vi "Random_Noise.vi"(9 "min":dbl, 10 "max":dbl, 11 "samples":i32) -> (3 "Random Noise":dbl[](array[numeric]))   [LabVIEW 2011]
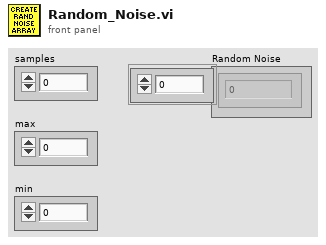
[diagram p1: front panel]
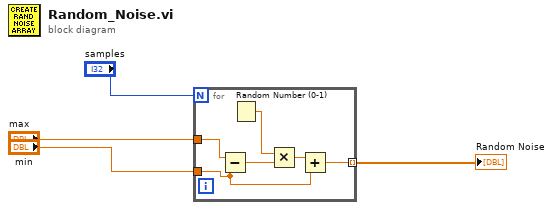
[diagram p0: block diagram]
diagram:
  n1 = for {
    N: "samples" -> [_]
    tunnel: "max" -> [w7]
    tunnel: "min" -> [w6]
    tunnel: [w5] -> w4 mode=indexing
    n2 = Subtract(x=w7, y=w6) -> (x-y=w9:dbl)
    n3 = Random Number (0-1)() -> (number: 0 to 1=w8:dbl)
    n4 = Multiply(x=w8, y=w9) -> (x*y=w10:dbl)
    n5 = Add(x=w10, y=w6) -> (x+y=w5:dbl)
  }
  "Random Noise" <- w4
